vi "Vision Processing.vi"(4 "error in (no error)":errorcluster) -> ()   [LabVIEW 2011]
doc: "This VI runs in parallel to other tasks. It gets images from the camera, processes them for color or shape and use that information to affect robot behavior."
uses:
  Robot Global Data.vi
  Global 1.vi
  <vilib>/vision/NI_Vision_Development_Module.lvlib
panel:
  in  "Camera Type":enum16{"206", "1011"}(ring)
  in  "Score Limits":T1={"Rect Coverage"=76.0, "Aspect Ratio"=70.0, "X Edge Strength"=40.0, "Y Edge Strength"=60.0}
  in  "Area Size Limit":i32=444
  in  "Particle Count Limit":i32=10
  out "Target Info":T2(array[cluster])
  in  "Processing":enum32{"Color", "Intensity", "Intensity Open"}(tab)
  in  "Luminance":i32=255
  in  "Saturation":i32=255
  in  "Hue":i32(knob)=65 scale=0.0..255.0
  in  "Margins":cluster{"Hue":i32, "Sat":i32, "Lum":i32}={"Hue"=9, "Sat"=40, "Lum"=19} {"Sat" scale=0.0..40.0; "Lum" scale=0.0..40.0; "Hue" scale=0.0..40.0}
  in  "Range":cluster{"Lower value":sgl, "Upper value":sgl}={"Lower value"=150.0, "Upper value"=255.0} {"Lower value" scale=0.0..255.0; "Upper value" scale=0.0..255.0}
  in  "Range 2":cluster{"Lower value":sgl, "Upper value":sgl}={"Lower value"=150.0, "Upper value"=255.0} {"Lower value" scale=0.0..255.0; "Upper value" scale=0.0..255.0}
  in  "Annotate":bool=TRUE
  out "Original Image":T3(plugin-control)
  out "Processed Image":T3(plugin-control)
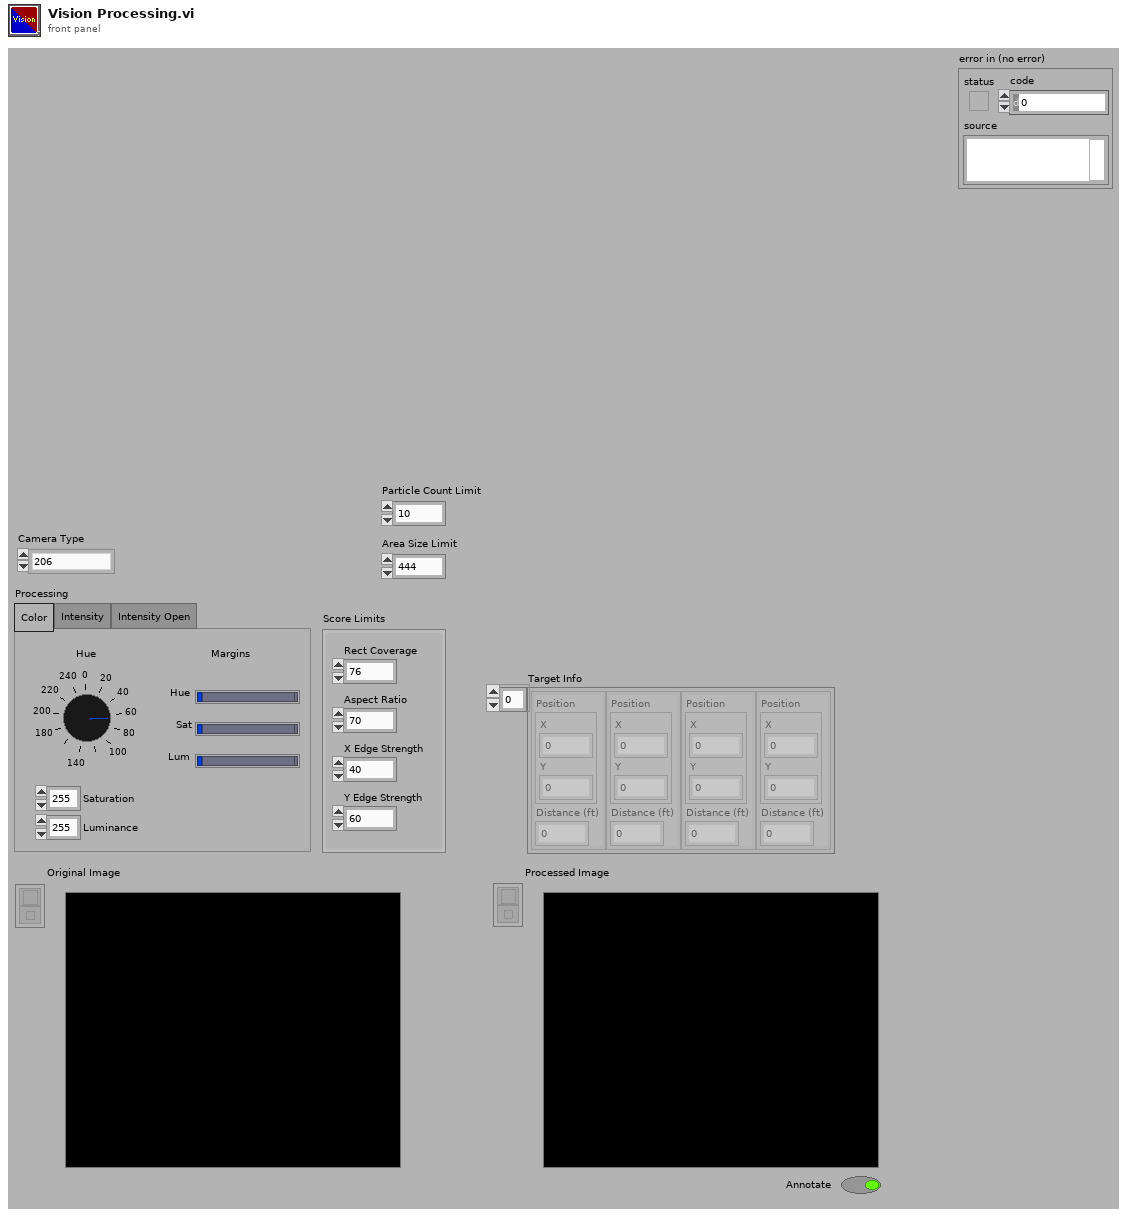
[diagram p1: front panel]
types:
  T1 = cluster{"Rect Coverage":dbl, "Aspect Ratio":dbl, "X Edge Strength":dbl, "Y Edge Strength":dbl}
  T2 = cluster{"Position":cluster{"X":dbl, "Y":dbl}, "Distance (ft)":dbl}[]
  T3 = typedef "IMAQ Image.ctl" = refnum<image>
  T4 = typedef "Image Type" = u32
  T5 = typedef "WPI_CameraDevRef.ctl" = cluster{"Camera Address":string, "CameraStatus":errorcluster, "Acquire Image Notifier":refnum<notifier>}
  T6 = enum32{"AutoM", "Close", "Dilate", "Erode", "Gradient", "Gradient out", "Gradient in", "Hit miss", "Open", "PClose", "POpen", "Thick", "Thin"}
  T7 = cluster{cluster{"Left":dbl, "Top":dbl, "Right":dbl, "Bottom":dbl}, dbl[]}[]
  T8 = cluster{"Left":dbl, "Top":dbl, "Right":dbl, "Bottom":dbl}
  T9 = cluster{"Target Center (-1 to 1)":cluster{"X":dbl, "Y":dbl}, "Distance (ft)":dbl}
  T10 = cluster{"Target Center (-1 to 1)":cluster{"X":dbl, "Y":dbl}, "Distance (ft)":dbl}[]
  T11 = typedef "WPI_CameraImageSize.ctl" = enum16{"640x480", "320x240", "160x120"}
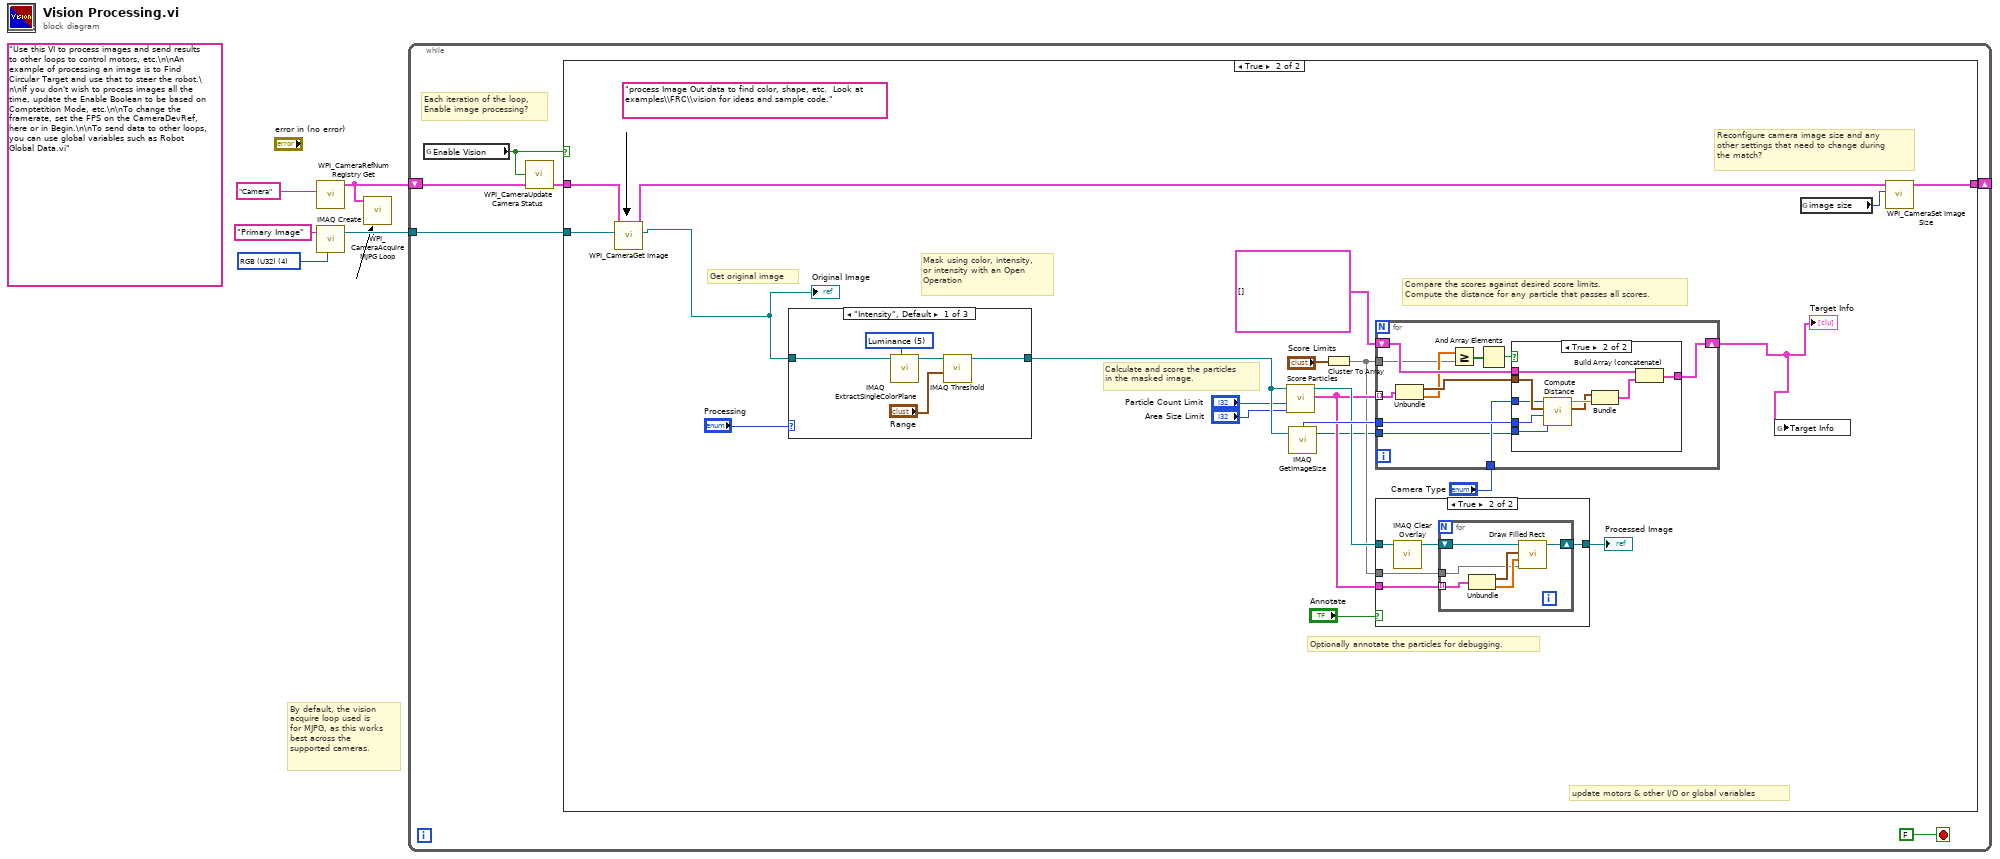
[diagram p0: block diagram]
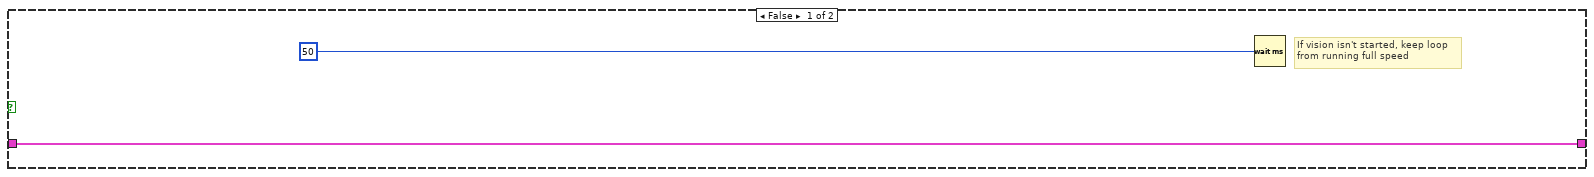
[diagram p2: hidden frame]
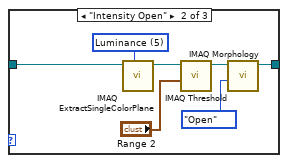
[diagram p4: hidden frame]
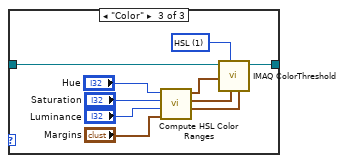
[diagram p5: hidden frame]
diagram:
  (unwired) "Use this VI to process images and send results to other loops to control motors, etc.\n\nAn example of processing an image is to Find Circular Target and use that to steer the robot.\n\nIf you don't wish to process images all the time, update the Enable Boolean to be based on Comptetition Mode, etc.\n\nTo change the framerate, set the FPS on the CameraDevRef, here or in Begin.\n\nTo send data to other loops, you can use global variables such as Robot Global Data.vi"
  w5 = T4 4 items=["Grayscale (U8)", "Grayscale (I16)", "Grayscale (SGL)", "Complex (CSG)", "RGB (U32)", "HSL (U32)", "RGB (U64)"] ("Image Type")
  # "By default, the vision\nacquire loop used is\nfor MJPG, as this works\nbest across the\nsupported cameras."
  n1 = call <vilib>:"WPI_CameraRefNum Registry Get.vi"("refnum name"="Camera") -> ("CameraDevRef"=w1:T5)  [unwired: 1 in, 9 out]
  n2 = call "IMAQ Create"("Image Name"="Primary Image", "Image Type"=w5) -> ("New Image"=w3:T3)  [unwired: 2 in, 2 out]
  n3 = call <vilib>:"WPI_CameraAcquire MJPG Loop.vi"("CameraDevRef"=w1) -> ()  [unwired: 11 in]
  n4 = while {
    shift-right: [w10] -> _
    shift-left: w1 -> [w8]
    tunnel: w3 -> [w9]
    stop <- FALSE stop-if-true
    # "Each iteration of the loop,\nEnable image processing?"
    n5 = global read "Robot Global Data.vi" "Enable Vision"() -> (w6:bool)
    n6 = call <vilib>:"WPI_CameraUpdate Camera Status.vi"("CameraDevRef In"=w8, "Enable Vision"=w6) -> ("CameraDevRef Out"=w7:T5)  [unwired: 3 in]
    n7 = case shown="True" w6 {
      tunnel: w9 -> [_ w33]
      tunnel: [w13 w34] -> w10
      tunnel: w7 -> [w13 w31]
      frame False {
        # "If vision isn't started, keep loop\nfrom running full speed"
        n8 = Wait (ms)(milliseconds to wait=u32 50) -> ()  [unwired: 1 out]
      }
      frame True {
        (unwired) "process Image Out data to find color, shape, etc.  Look at examples\\FRC\\vision for ideas and sample code."
        # "Optionally annotate the particles for debugging."
        # "Compare the scores against desired score limits.\nCompute the distance for any particle that passes all scores."
        # "Calculate and score the particles\nin the masked image."
        # "Mask using color, intensity,\nor intensity with an Open\nOperation"
        # "Get original image"
        # "update motors & other I/O or global variables"
        # "Reconfigure camera image size and any\nother settings that need to change during\nthe match?"
        n9 = call <vilib>:"WPI_CameraGet Image.vi"("Image"=w33, "CameraDevRef"=w31) -> ("Image Out"=w29:T3, "CameraDevRef Out"=w30:T5)  [unwired: 1 in, 7 out]
        "Original Image" <- w29
        n10 = case shown="\"Intensity\", Default" "Processing" {
          tunnel: w29 -> [w51 w58 w68]
          tunnel: [w48 w53 w67] -> w19
          frame "Intensity", Default {
            w47 = 5 items=["Red", "Green", "Blue", "Hue", "Saturation", "Luminance", "Value", "Intensity"] ("Color Plane")
            n11 = call "IMAQ ExtractSingleColorPlane"("Color Plane"=w47, "Image Src"=w51) -> ("Image Dst Out"=w50:T3)  [unwired: 2 in, 7 out]
            n12 = call "IMAQ Threshold"("Range"="Range", "Image Src"=w50) -> ("Image Dst Out"=w48:T3)  [unwired: 4 in, 5 out]
          }
          frame "Intensity Open" {
            w52 = 5 items=["Red", "Green", "Blue", "Hue", "Saturation", "Luminance", "Value", "Intensity"] ("Color Plane")
            n13 = call "IMAQ ExtractSingleColorPlane"("Color Plane"=w52, "Image Src"=w58) -> ("Image Dst Out"=w57:T3)  [unwired: 2 in, 7 out]
            n14 = call "IMAQ Threshold"("Range"="Range 2", "Image Src"=w57) -> ("Image Dst Out"=w54:T3)  [unwired: 4 in, 5 out]
            n15 = call "IMAQ Morphology"("Operation"=T6."Open", "Image Src"=w54) -> ("Image Dst Out"=w53:T3)  [unwired: 8 in, 1 out]
          }
          frame "Color" {
            w66 = u16 1 items=["RGB", "HSL", "HSV", "HSI"] ("Color Mode")
            n16 = call "Compute HSL Color Ranges.vi"("Margins"="Margins", "Luminance"="Luminance", "Saturation"="Saturation", "Hue"="Hue") -> ("Lum Range"=w63:cluster{i32, i32}, "Sat Range"=w64:cluster{i32, i32}, "Hue Range"=w65:cluster{i32, i32})  [unwired: 5 in]
            n17 = call "IMAQ ColorThreshold"("Blue or Luma or Val or Inten Range"=w63, "Green or Sat Range"=w64, "Color Mode"=w66, "Red or Hue Range"=w65, "Image Src"=w68) -> ("Image Dst Out"=w67:T3)  [unwired: 5 in, 1 out]
          }
        }
        n18 = call "Score Particles.vi"("Area Size Limit"="Area Size Limit", "Particle Count Limit"="Particle Count Limit", "Image Refnum in"=w19) -> ("Scored Particle Info"=w22:T7, "Image Refnum out"=w26:T3)  [unwired: 7 in]
        n19 = call "IMAQ GetImageSize"("Image"=w19) -> ("Y Resolution"=w15:i32, "X Resolution"=w27:i32)  [unwired: 3 in, 1 out]
        n20 = Cluster To Array(cluster="Score Limits") -> (array=w20:dbl[])
        n21 = for {
          shift-right: [w78] -> w14
          shift-left: T2 [] -> [w79]
          tunnel: w27 -> [w77]
          tunnel: w22 -> [w75] mode=indexing
          tunnel: w20 -> [w70]
          tunnel: "Camera Type" -> [w74]
          tunnel: w15 -> [w69]
          n22 = Unbundle(w75) -> (w76:T8, w71:dbl[])
          n23 = Greater Or Equal?(x=w71, y=w70) -> (x >= y?=w73:bool[])
          n24 = And Array Elements(Boolean array=w73) -> (logical AND=w72:bool)
          n25 = case shown="True" w72 {
            tunnel: w79 -> [w80 w89]
            tunnel: [w80 w88] -> w78
            tunnel: w76 -> [_ w84]
            tunnel: w77 -> [_ w86]
            tunnel: w74 -> [_ w83]
            tunnel: w69 -> [_ w81]
            frame False {
            }
            frame True {
              n26 = call "Compute Distance.vi"("Y Image Resolution"=w81, "X Image Resolution"=w86, "Bounding Box"=w84, "Camera Type"=w83) -> ("Target Center (-1 to 1)"=w82:cluster{"X":dbl, "Y":dbl}, "Distance (ft)"=w85:dbl)  [unwired: 6 in]
              n27 = Bundle("Target Center (-1 to 1)"=w82, "Distance (ft)"=w85) -> (w87:T9)  [unwired: 1 in]
              n28 = Build Array (concatenate)(w89, w87) -> (w88:T10)
            }
          }
        }
        "Target Info" <- w14
        n29 = case shown="True" "Annotate" {
          tunnel: w26 -> [w35 w40]
          tunnel: [w35 w39] -> w23
          tunnel: w22 -> [_ w37]
          tunnel: w20 -> [_ w36]
          frame False {
          }
          frame True {
            n30 = call "IMAQ Clear Overlay"("Image"=w40) -> ("Image Out"=w38:T3)  [unwired: 2 in, 8 out]
            n31 = for {
              shift-right: [w45] -> w39
              shift-left: w38 -> [w46]
              tunnel: w37 -> [w42] mode=indexing
              tunnel: w36 -> [w41]
              n32 = Unbundle(w42) -> (w43:T8, w44:dbl[])
              n33 = call "Draw Filled Rect.vi"("Limits"=w41, "Scores"=w44, "Bounding Box"=w43, "image in"=w46) -> ("image out"=w45:T3)  [unwired: 7 in]
            }
          }
        }
        "Processed Image" <- w23
        n34 = global write "Global 1.vi" "Target Info"(w14) -> ()
        n35 = global read "Robot Global Data.vi" "image size"() -> (w32:T11)
        n36 = call <vilib>:"WPI_CameraSet Image Size.vi"("Image Size"=w32, "CameraDevRef"=w30) -> ("CameraDevRef Out"=w34:T5)  [unwired: 1 in, 8 out]
      }
    }
  }
